vi "Set Channel.vi"(0 "CS.lvclass in":refnum<class "CS.lvclass">, 5 "Channel":u8, 7 "I&R In":T1 {"Current" min=0.0}, 11 "error in (no error)":errorcluster) -> (4 "CS.lvclass out":refnum<class "CS.lvclass">, 15 "error out":errorcluster)   [LabVIEW 2013, in "CS.lvclass"]
uses:
  Lib.llb/CS.lvclass
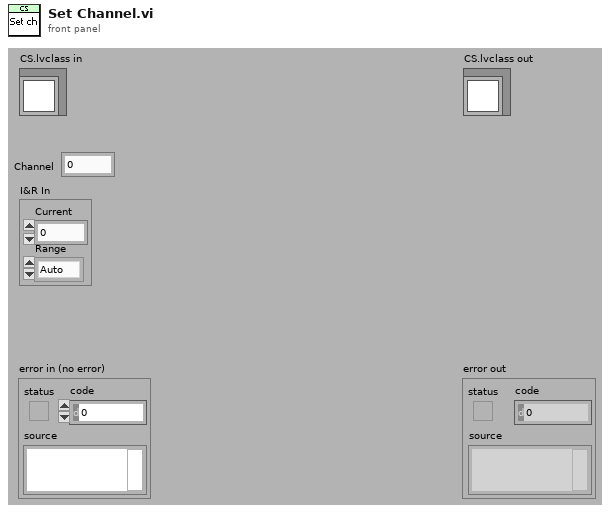
[diagram p1: front panel]
types:
  T1 = cluster{"Current":dbl, "Range":enum8{"Auto", "x1 uA", "x10 uA", "x100 uA", "x1 mA"}}
  T2 = enum8{"Auto", "x1 uA", "x10 uA", "x100 uA", "x1 mA"}
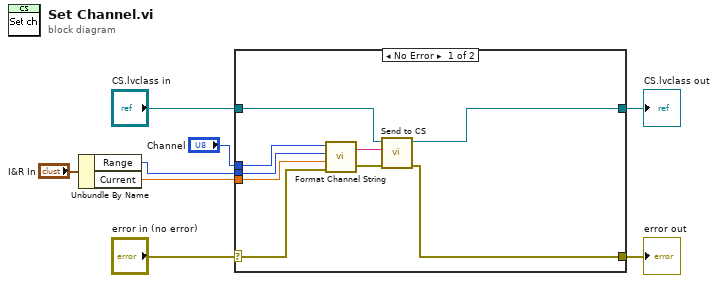
[diagram p0: block diagram]
diagram:
  n1 = Unbundle By Name("I&R In") -> ("Range"=w2:T2, "Current"=w1:dbl)
  n2 = case shown="No Error" "error in (no error)" {
    selector: "error in (no error)" -> [w17 w18]
    tunnel: [w9 w18] -> w7
    tunnel: [w12 w19] -> w5
    tunnel: "CS.lvclass in" -> [w13 w19]
    tunnel: "Channel" -> [w16 _]
    tunnel: w2 -> [w15 _]
    tunnel: w1 -> [w14 _]
    frame No Error {
      n3 = call "Format Channel String.vi"("error IO 2"=w17, "Current"=w14, "Range"=w15, "Channel"=w16) -> ("error IO"=w10:errorcluster, "String"=w11:string)
      n4 = call-dynamic "Send to CS.vi"("error in (no error)"=w10, "String to write"=w11, "CS in"=w13) -> ("error out"=w9:errorcluster, "CS out"=w12:refnum<class "CS.lvclass">)  [unwired: 7 in]
    }
    frame Error {
    }
  }
  "error out" <- w7
  "CS.lvclass out" <- w5
